vi "Get SMO Port.vi"(8 "error in (no error)":errorcluster, 11 "instrument.OptiCool in":refnum<class "instrument.OptiCool.lvclass">) -> (0 "error out":errorcluster, 2 "Port":u16, 3 "instrument.OptiCool out":refnum<class "instrument.OptiCool.lvclass">)   [LabVIEW 2019, in "instrument.OptiCool.lvclass"]
uses:
  instrument.OptiCool.lvclass
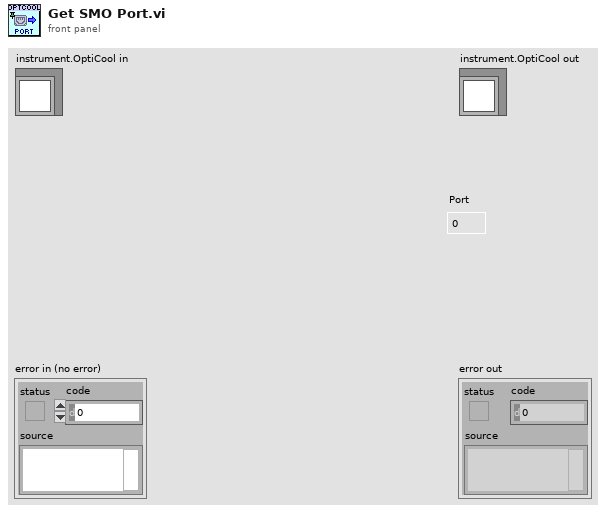
[diagram p1: front panel]
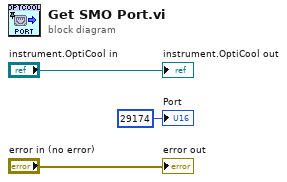
[diagram p0: block diagram]
diagram:
  "error out" <- "error in (no error)"
  "instrument.OptiCool out" <- "instrument.OptiCool in"
  "Port" <- u16 29174 ("Port")
